vi "sync_shutter.vi"(1 "Do acquire?":bool, 2 "Old acquire state":bool, 3 "Sync shutter to acquisition":bool, 4 "Control_Shutter_Queue":refnum<queue>) -> ()   [LabVIEW 2010]
uses:
  typedefs/control_shutter_enum.ctl
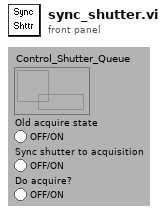
[diagram p1: front panel]
types:
  T1 = typedef "control_shutter_enum.ctl" = enum16{"Init", "Open", "Close", "Quit"}
  T2 = cluster{"Control shutter enum":T1, "variant":variant}
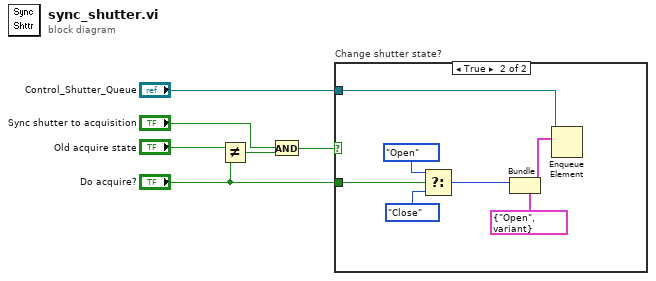
[diagram p0: block diagram]
diagram:
  n1 = Not Equal?(x="Old acquire state", y="Do acquire?") -> (x != y?=w2:bool)
  n2 = And(x="Sync shutter to acquisition", y=w2) -> (x .and. y?=w4:bool)
  n3 = case "Change shutter state?" shown="True" w4 {
    tunnel: "Control_Shutter_Queue" -> [_ w13]
    tunnel: "Do acquire?" -> [_ w12]
    frame False {
    }
    frame True {
      n4 = Select(t=control_shutter_enum."Open" ("Control shutter enum"), s=w12, f=control_shutter_enum."Close" ("Control shutter enum")) -> (s? t:f=w8:T1)
      n5 = Bundle(cluster=T2 {"Control shutter enum"=enum."Open", "variant"=variant} ("element"), "Control shutter enum"=w8) -> (w7:T2)  [unwired: 1 in]
      n6 = Enqueue Element(queue=w13, element=w7) -> ()  [unwired: 2 in, 3 out]
    }
  }
